vi "Write Pulse Width.vi"(8 "error in":errorcluster, 10 "Pulse Width":dbl, 11 "Electronic Load in":refnum<class "Electronic Load.lvclass">) -> (0 "error out":errorcluster, 3 "Electronic Load out":refnum<class "Electronic Load.lvclass">)   [LabVIEW 2019, in "Electronic Load.lvlib" / "Electronic Load.lvclass"]
uses:
  Library/Electronic Load.lvclass
  C:/Users/Public/Documents/Development/builds/Instruments/Instruments.lvlibp/Library/Instruments.lvclass
  Library/Electronic Load.lvclass/Electronic Load.ctl
  builds/Instruments/Instruments.lvlibp/Private/Polymorphic/Integers/Event from DBL.vi
  builds/Instruments/Instruments.lvlibp/Accessors/Command with Logging.vi
  builds/Instruments/Instruments.lvlibp/Library/Instruments.lvclass
  builds/Instruments/Instruments.lvlibp
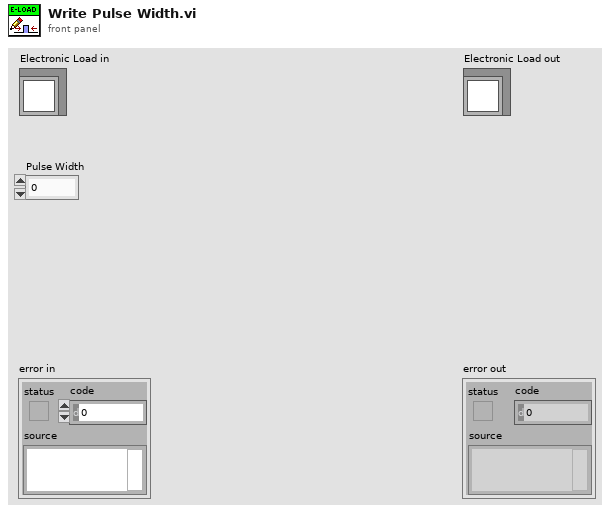
[diagram p1: front panel]
types:
  T1 = cluster{"Timestamp":timestamp, "Description":string, "Data":string}
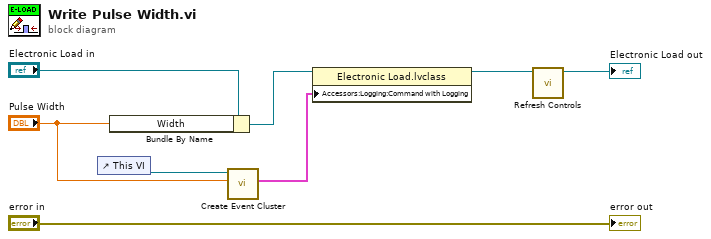
[diagram p0: block diagram]
diagram:
  n1 = control-ref of="This VI"() -> (w7:refnum<vi>)
  n2 = Bundle By Name(cluster="Electronic Load in", "Width"="Pulse Width") -> (w4:refnum<class "Electronic Load.lvclass">)
  n3 = call-poly "Create Event Cluster.vi"("Value"="Pulse Width", "VI Refnum"=w7) -> ("Event Data"=w6:T1)  [unwired: 9 in]
  n4 = property class="Electronic Load.lvclass"(reference=w4, "Accessors:Logging:Command with Logging"=w6) -> (reference out=w2:refnum<class "Electronic Load.lvclass">)  [unwired: 1 in, 1 out]
  n5 = call "Refresh Controls.vi"("Electronic Load in"=w2) -> ("Electronic Load out"=→"Electronic Load out":refnum<class "Electronic Load.lvclass">)  [unwired: 9 in, 1 out]
  "error out" <- "error in"
